vi "TimeCalculation.vi"(5 "Speed Z":i32, 7 "Position Z":i32, 8 "SpeedY":i32, 9 "Y Position":i32, 10 "Speed X":i32, 11 "X Position":i32) -> (3 "Time":dbl)   [LabVIEW 2017]
uses:
  Settings/Traverse-Settings-Global.vi
panel:
  out "x*y":dbl
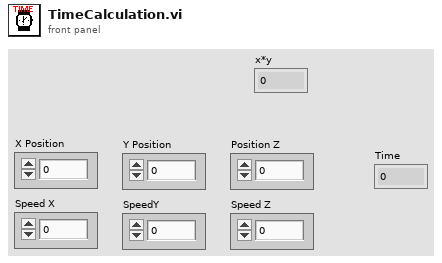
[diagram p1: front panel]
types:
  T1 = typedef "Settings-Control.ctl" = cluster{"Acceleration":dbl[], "Deceleration":dbl[], "Max Velocity":dbl[], "Speed":dbl, "Pulse/Degree":dbl, "Degre Factor":dbl[], "mm/rotation":dbl[], "Traverse Name":string}
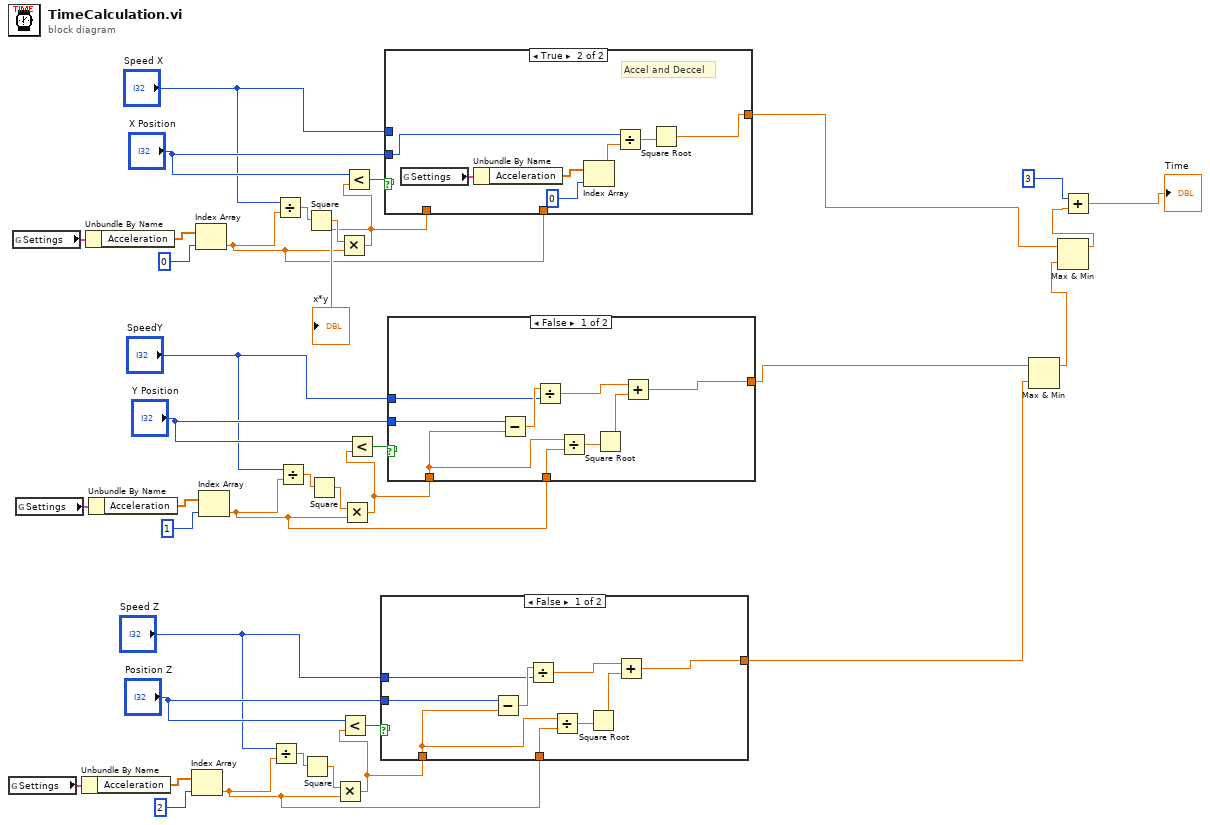
[diagram p0: block diagram]
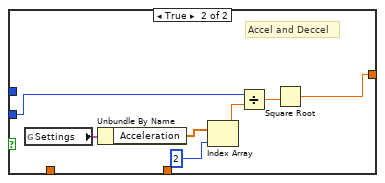
[diagram p2: hidden frame]
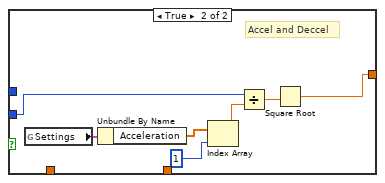
[diagram p3: hidden frame]
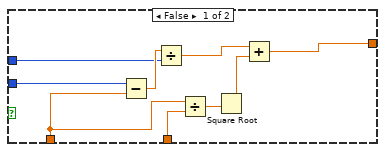
[diagram p4: hidden frame]
diagram:
  n1 = global read "Traverse-Settings-Global.vi" "Settings"() -> (w17:T1)
  n2 = global read "Traverse-Settings-Global.vi" "Settings"() -> (w35:T1)
  n3 = global read "Traverse-Settings-Global.vi" "Settings"() -> (w26:T1)
  n4 = Unbundle By Name(w17) -> ("Acceleration"=w16:dbl[])
  n5 = Unbundle By Name(w35) -> ("Acceleration"=w34:dbl[])
  n6 = Unbundle By Name(w26) -> ("Acceleration"=w25:dbl[])
  n7 = Index Array(array=w16, index=2) -> (element=w11:dbl)
  n8 = Index Array(array=w34, index=0) -> (element=w29:dbl)
  n9 = Index Array(array=w25, index=1) -> (element=w20:dbl)
  n10 = Divide(x="Speed Z", y=w11) -> (x/y=w14:dbl)
  n11 = Divide(x="Speed X", y=w29) -> (x/y=w32:dbl)
  n12 = Divide(x="SpeedY", y=w20) -> (x/y=w23:dbl)
  n13 = Square(x=w14) -> (x^2=w13:dbl)
  n14 = Square(x=w32) -> (x^2=w31:dbl)
  n15 = Square(x=w23) -> (x^2=w22:dbl)
  n16 = Multiply(x=w13, y=w11) -> (x*y=w12:dbl)
  n17 = Multiply(x=w31, y=w29) -> (x*y=w30:dbl)
  "x*y" <- w30
  n18 = Less?(x="Position Z", y=w12) -> (x < y?=w18:bool)
  n19 = Multiply(x=w22, y=w20) -> (x*y=w21:dbl)
  n20 = Less?(x="X Position", y=w30) -> (x < y?=w36:bool)
  n21 = Less?(x="Y Position", y=w21) -> (x < y?=w27:bool)
  n22 = case shown="False" w18 {
    tunnel: "Position Z" -> [w46 w47]
    tunnel: "Speed Z" -> [w44 _]
    tunnel: [w43 w48] -> w8
    tunnel: w12 -> [w40 _]
    tunnel: w11 -> [w39 _]
    frame False {
      n23 = Subtract(x=w46, y=w40) -> (x-y=w45:dbl)
      n24 = Divide(x=w45, y=w44) -> (x/y=w42:dbl)
      n25 = Divide(x=w40, y=w39) -> (x/y=w41:dbl)
      n26 = Square Root(x=w41) -> (sqrt(x)=w38:dbl)
      n27 = Add(x=w42, y=w38) -> (x+y=w43:dbl)
    }
    frame True {
      # "Accel and Deccel"
      n28 = global read "Traverse-Settings-Global.vi" "Settings"() -> (w53:T1)
      n29 = Unbundle By Name(w53) -> ("Acceleration"=w52:dbl[])
      n30 = Index Array(array=w52, index=2) -> (element=w50:dbl)
      n31 = Divide(x=w47, y=w50) -> (x/y=w49:dbl)
      n32 = Square Root(x=w49) -> (sqrt(x)=w48:dbl)
    }
  }
  n33 = case shown="True" w36 {
    tunnel: "X Position" -> [w62 w63]
    tunnel: "Speed X" -> [w60 _]
    tunnel: [w59 w64] -> w5
    tunnel: w30 -> [w56 _]
    tunnel: w29 -> [w55 _]
    frame False {
      n34 = Subtract(x=w62, y=w56) -> (x-y=w61:dbl)
      n35 = Divide(x=w61, y=w60) -> (x/y=w58:dbl)
      n36 = Divide(x=w56, y=w55) -> (x/y=w57:dbl)
      n37 = Square Root(x=w57) -> (sqrt(x)=w54:dbl)
      n38 = Add(x=w58, y=w54) -> (x+y=w59:dbl)
    }
    frame True {
      # "Accel and Deccel"
      n39 = global read "Traverse-Settings-Global.vi" "Settings"() -> (w69:T1)
      n40 = Unbundle By Name(w69) -> ("Acceleration"=w68:dbl[])
      n41 = Index Array(array=w68, index=0) -> (element=w66:dbl)
      n42 = Divide(x=w63, y=w66) -> (x/y=w65:dbl)
      n43 = Square Root(x=w65) -> (sqrt(x)=w64:dbl)
    }
  }
  n44 = case shown="False" w27 {
    tunnel: "Y Position" -> [w78 w79]
    tunnel: "SpeedY" -> [w76 _]
    tunnel: [w75 w80] -> w7
    tunnel: w21 -> [w72 _]
    tunnel: w20 -> [w71 _]
    frame False {
      n45 = Subtract(x=w78, y=w72) -> (x-y=w77:dbl)
      n46 = Divide(x=w77, y=w76) -> (x/y=w74:dbl)
      n47 = Divide(x=w72, y=w71) -> (x/y=w73:dbl)
      n48 = Square Root(x=w73) -> (sqrt(x)=w70:dbl)
      n49 = Add(x=w74, y=w70) -> (x+y=w75:dbl)
    }
    frame True {
      # "Accel and Deccel"
      n50 = global read "Traverse-Settings-Global.vi" "Settings"() -> (w85:T1)
      n51 = Unbundle By Name(w85) -> ("Acceleration"=w84:dbl[])
      n52 = Index Array(array=w84, index=1) -> (element=w82:dbl)
      n53 = Divide(x=w79, y=w82) -> (x/y=w81:dbl)
      n54 = Square Root(x=w81) -> (sqrt(x)=w80:dbl)
    }
  }
  n55 = Max & Min(x=w7, y=w8) -> (max(x,y)=w6:dbl)  [unwired: 1 out]
  n56 = Max & Min(x=w5, y=w6) -> (max(x,y)=w9:dbl)  [unwired: 1 out]
  n57 = Add(x=3, y=w9) -> (x+y=→"Time":dbl)
